vi "GetAlazar_SynthFocus_25_GPU - ATS-SDK.vi"(1 "Digitizer Settings":T4={"Digitizer delay (us) "=0.0, "rf points per line"=2048, "lines per plane"=128, "Samp Rate (Hz)"=100000000.0, "Additional dig delay (us)"=0.0, "Voltage Scale"=0.4, "Pre-Looks"=0, "Offset delay (us)"=0.0, "bits A/D"=8, "Avg Num"=1, "DigTimeOut"=5.0, "Rel Dig Delay"=0.0, "Dig Ch"=0, "LeCroyCluster"={"LeCroy Channels"=[TRUE, FALSE, FALSE, FALSE], "LC read pt offset"=0.0, "Sweep Avg"=FALSE}, "Main Digitizer"=enum."NI Digitizer", "Dig Config"=enum."Single channel", "Digitizer ID Cluster"={"Acqiris/Alazar/SP ID"=[], "NI Instr Handles"=[], "LeCroy VISA"="", "GaGe Handle"={"Handle"=0, "Sample size"=0, "Resolution"=0, "Offset"=0, "Channels"=0, "Boards"=0}, "ATS Ref"="ATS9350", "Acqiris Address"=["PCI::INSTR0"], "ADQRef"=refnum, "adq_cu_ptr"=refnum}, "Trigger Settings"={"Trig Source"=1, "Trig Coupling"=0, "Trig Slope"=0, "Level (mV)"=1500.0}, "Bulk Acq"=FALSE, "Bulk Start Indexes"=[], "Data Ref RF"=refnum, "NI ID/Channel"=[], "Total Dig CH"=1, "Xtra Ann Trig delay (us)"=10.0, "Fix Z Delay?"=FALSE, "One Way Transmission?"=FALSE, "Data Ref Log"=refnum} {"Trigger Settings"."Trig Slope" items=["Positive", "Negative"]; "Trigger Settings"."Level (mV)" format="%.2f"; "Trigger Settings"."Trig Coupling" items=["DC 1 MOhm", "AC 1 MOhm", "DC 50 Ohm", "AC 50 Ohm"]; "Trigger Settings"."Trig Source" items=["Chan 1", "External"]; "Rel Dig Delay" format="%.2f"; "DigTimeOut" format="%.2f"; "Avg Num" min=1; "Offset delay (us)" format="%.2f"; "Additional dig delay (us)" format="%.2f"; "Digitizer delay (us)" format="%.2f"}, 2 "AlazarCluster":T8, 5 "errorin":errorcluster, 7 "Ann Array Params":T1={"Synth Foc?"=FALSE, "Focal Zones"=41, "Switch T/R"=0, "Trans Geometry (mm)"={"Transducer"=0, "Geo Focus"=12.0, "a (radius)"=3.0, "# of rings"=5, "kerf space "=0.1, "Center Freq"=12.0}, "Sub Ap Excite?"=FALSE, "Full Array Scan?"=FALSE, "Xmt/Rcv"={"XMIT"=[TRUE, TRUE, TRUE, TRUE, TRUE], "RCV"=[TRUE, TRUE, TRUE, TRUE, TRUE]}, "PulseSpacing (us)"=0.0, "Xmit Ring"=0, "XMIT CHS"=0, "RCV CHS"=0, "GPU?"=FALSE, "Save TIFF?"=FALSE, "downfactor"=1, "RCV 1CH"=0} {"RCV 1CH" items=["All", "1", "2", "3", "4", "5"]; "Trans Geometry (mm)"."Transducer" items=["6D 12R 40 MHz"=0, "10D 31R 20 MHz"=1, "10D 23R 20 MHz"=2, "6D 23R 40 MHz"=3, "4.5D 10.7R 40 MHz"=4, "9D 23.5R 20 MHz"=5, "9D 25.8R 20MHz"=6, "Enter"=99]; "Switch T/R" min=1 max=5 step=1}, 8 "lines per plane":i32, 11 "Reverse?":bool) -> (12 "Gain Array":T9(array[cluster]), 13 "Raw VGain (scale)":dbl, 15 "VGain (dB)":dbl, 19 "error out":errorcluster)   [LabVIEW 2022 SP3]
uses:
  -DigitizerRoutines/DigitizerSettings.ctl
  -DigitizerRoutines/Digitizer.ctl
  -DigitizerRoutines/DigConfig.ctl
  -DigitizerRoutines/DigitizerID.ctl
  C:/Windows/System32/ADQAPI_dotNet_helper.dll
  Windows/System32/ADQAPI_dotNet_helper.dll
  Annular Array/-AnnularRoutines/AnnularArray.ctl
  Annular Array/-AnnularRoutines/TransGeometry.ctl
  Annular Array/-AnnularRoutines/ArrayGeometry.ctl
panel:
  out "read time":u32
  out "Synth focus time time":u32
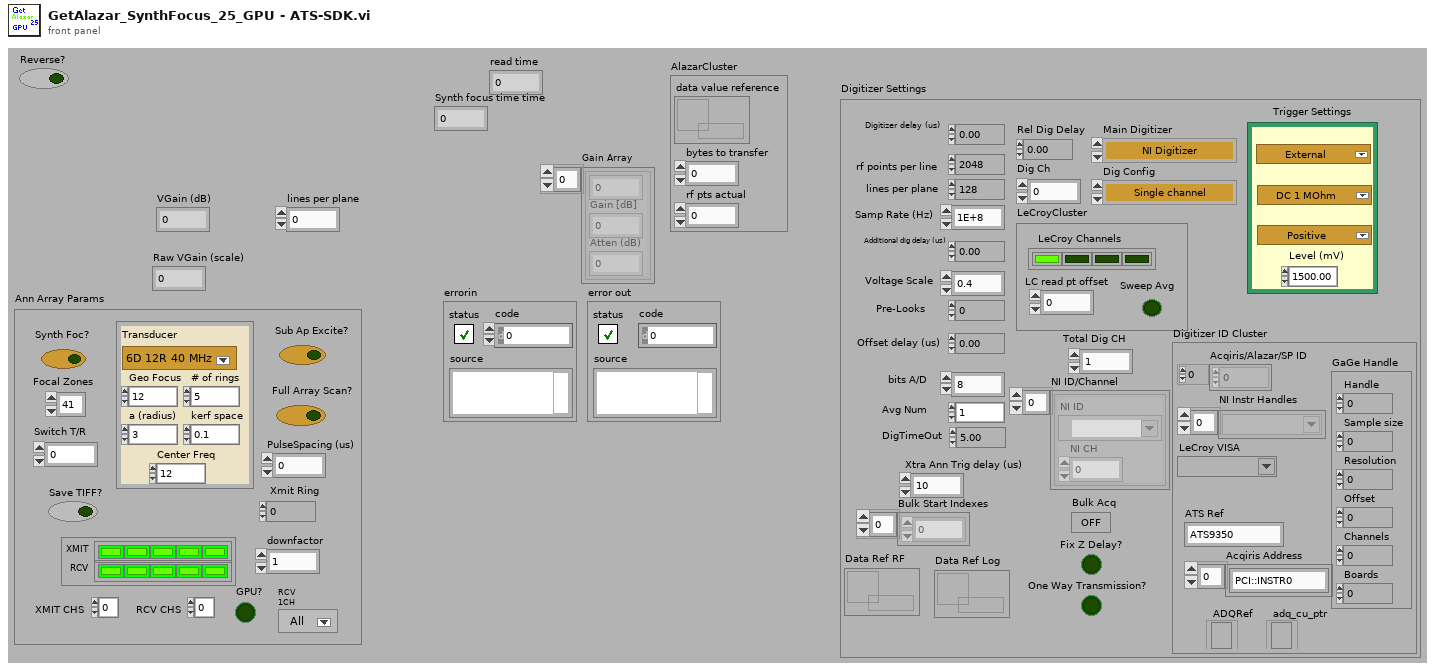
[diagram p1: front panel]
types:
  T1 = typedef "AnnularArray.ctl" = cluster{"Synth Foc?":bool, "Focal Zones":i16, "Switch T/R":i16, "Trans Geometry (mm)":T2, "Sub Ap Excite?":bool, "Full Array Scan?":bool, "Xmt/Rcv":cluster{"XMIT":bool[], "RCV":bool[]}, "PulseSpacing (us)":sgl, "Xmit Ring":i32, "XMIT CHS":u8, "RCV CHS":u8, "GPU?":bool, "Save TIFF?":bool, "downfactor":i32, "RCV 1CH":u16}
  T2 = typedef "TransGeometry.ctl" = cluster{"Transducer":T3, "Geo Focus":dbl, "a (radius)":dbl, "# of rings":i32, "kerf space ":dbl, "Center Freq":dbl}
  T3 = typedef "ArrayGeometry.ctl" = u16
  T4 = typedef "DigitizerSettings.ctl" = cluster{"Digitizer delay (us) ":dbl, "rf points per line":i32, "lines per plane":i32, "Samp Rate (Hz)":dbl, "Additional dig delay (us)":dbl, "Voltage Scale":dbl, "Pre-Looks":i32, "Offset delay (us)":dbl, "bits A/D":i8, "Avg Num":i32, "DigTimeOut":sgl, "Rel Dig Delay":sgl, "Dig Ch":i32, "LeCroyCluster":cluster{"LeCroy Channels":bool[], "LC read pt offset":dbl, "Sweep Avg":bool}, "Main Digitizer":T5, "Dig Config":T6, "Digitizer ID Cluster":T7, "Trigger Settings":cluster{"Trig Source":u16, "Trig Coupling":u16, "Trig Slope":u16, "Level (mV)":dbl}, "Bulk Acq":bool, "Bulk Start Indexes":i32[], "Data Ref RF":refnum<data-value>, "NI ID/Channel":cluster{"NI ID":refnum<k15>, "NI CH":i32}[], "Total Dig CH":i32, "Xtra Ann Trig delay (us)":dbl, "Fix Z Delay?":bool, "One Way Transmission?":bool, "Data Ref Log":refnum<data-value>}
  T5 = typedef "Digitizer.ctl" = enum16{"Acqiris Digitizer", "NI Digitizer", "LeCroy", "GaGe", "AlazarTech", "No Digitizer", "Teledyne"}
  T6 = typedef "DigConfig.ctl" = enum16{"Single channel", "2 Chans w/ 2 Acqiris", "2 Chans w/ 1 Acqiris", "5-CH Pulser New", "5-CH pulser w/ ann array", "5-pass style ann array", "Empty"}
  T7 = typedef "DigitizerID.ctl" = cluster{"Acqiris/Alazar/SP ID":u32[], "NI Instr Handles":refnum<k15>[], "LeCroy VISA":refnum<visa-resource-name>, "GaGe Handle":cluster{"Handle":u32, "Sample size":u32, "Resolution":i32, "Offset":i32, "Channels":u32, "Boards":u32}, "ATS Ref":string, "Acqiris Address":string[], "ADQRef":refnum<k24>, "adq_cu_ptr":refnum<k24>}
  T8 = cluster{"data value reference":refnum<data-value>, "bytes to transfer":u32, "rf pts actual":u32}
  T9 = cluster{sgl, "Gain [dB]  ":sgl, "Atten (dB)":sgl}[]
  T10 = cluster{sgl, "Gain [dB]  ":sgl, "Atten (dB)":sgl}
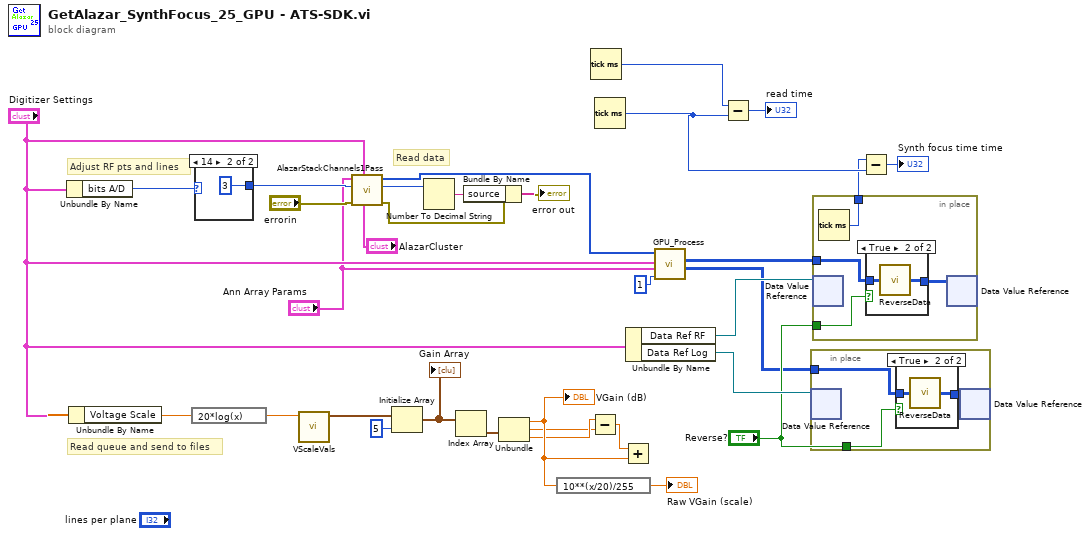
[diagram p0: block diagram]
diagram:
  # "Read data"
  # "Adjust RF pts and lines"
  # "Read queue and send to files"
  n1 = Unbundle By Name("Digitizer Settings") -> ("bits A/D"=w21:i8)
  n2 = Unbundle By Name("Digitizer Settings") -> ("Voltage Scale"=w22:dbl)
  n3 = expression code="20*log(x)"(w22) -> (w24:dbl)
  n4 = case shown="14" w21 {
    tunnel: [_ u16 3 ("Extra Shift")] -> w3
    frame 0, Default {
    }
    frame 14 {
    }
  }
  n5 = call "VScaleVals.vi"("Full Scale"=w24) -> ("Voltage Scale"=w15:T10)  [unwired: 8 in, 2 out]
  n6 = call "AlazarStackChannels1Pass.vi"("AlazarCluster"="AlazarCluster", "Digitizer Settings"="Digitizer Settings", "error in"="errorin", "Extra Shift"=w3, "Ann Array Params"="Ann Array Params") -> ("error out"=w8:errorcluster, "Return Code"=w6:u32, "DataInterleavedOut"=w2:i16[])  [unwired: 2 in, 2 out]
  n7 = Initialize Array(w15, 5 ("dimension size")) -> (w13:T9)
  "Gain Array" <- w13
  n8 = Number To Decimal String(number=w6) -> (decimal integer string=w23:string)  [unwired: 1 in]
  n9 = Index Array(array=w13) -> (element=w33:T10)  [unwired: 1 in]
  n10 = Bundle By Name(cluster=w8, "source"=w23) -> (→"error out":errorcluster)
  n11 = Unbundle(w33) -> (w32:sgl, "Gain [dB]"=w30:sgl, "Atten (dB)"=w31:sgl)
  "VGain (dB)" <- w32
  n12 = expression code="10**(x/20)/255"(w32) -> (→"Raw VGain (scale)":sgl)
  n13 = Subtract(x=w31, y=w30) -> (x-y=w29:sgl)
  n14 = Tick Count (ms)() -> (millisecond timer value=w10:u32)
  n15 = Tick Count (ms)() -> (millisecond timer value=w27:u32)
  n16 = Add(x=w29, y=w32) -> ()  [unwired: 1 out]
  n17 = Unbundle By Name("Digitizer Settings") -> ("Data Ref RF"=w19:refnum<data-value>, "Data Ref Log"=w18:refnum<data-value>)
  n18 = call "GPU_Process.vi"("DataFlag"=1, "Ann Array Params"="Ann Array Params", "Digitizer Settings"="Digitizer Settings", "Raw Data In"=w2) -> ("RFimageData"=w11:i16[][], "RF_Out"=w12:i16[][])  [unwired: 5 in, 1 out]
  n19 = Subtract(x=w10, y=w27) -> (x-y=→"read time":u32)
  n20 = in-place {
    in-place-border: w11 -> [w36]
    in-place-border: "Reverse?" -> [w35]
    n21 = in-place-dvr #1(w18) -> ()  [unwired: 2 out]
    n22 = case shown="True" w35 {
      tunnel: w36 -> [w38 w40]
      tunnel: [w38 w39] -> w37
      frame False {
      }
      frame True {
        n23 = call "ReverseData.vi"("Array in"=w40) -> ("Array out"=w39:i16[][])
      }
    }
    n24 = in-place-dvr #1(w37) -> ()  [unwired: 2 out]
  }
  n25 = in-place {
    in-place-border: w12 -> [w42]
    in-place-border: [w44] -> w17
    in-place-border: "Reverse?" -> [w41]
    n26 = in-place-dvr #2(w19) -> ()  [unwired: 2 out]
    n27 = Tick Count (ms)() -> (millisecond timer value=w44:u32)
    n28 = case shown="True" w41 {
      tunnel: w42 -> [w45 w47]
      tunnel: [w45 w46] -> w43
      frame False {
      }
      frame True {
        n29 = call "ReverseData.vi"("Array in"=w47) -> ("Array out"=w46:i16[][])
      }
    }
    n30 = in-place-dvr #2(w43) -> ()  [unwired: 2 out]
  }
  n31 = Subtract(x=w17, y=w27) -> (x-y=→"Synth focus time time":u32)
